vi "CurrentTaskName Request.vi"(8 "error in (no error)":errorcluster, 11 "BuildWorker in":refnum<class "BuildWorker.lvclass">) -> (0 "error out":errorcluster, 3 "BuildWorker out":refnum<class "BuildWorker.lvclass">)   [LabVIEW 2017, in "BuildWorker.lvlib" / "BuildWorker.lvclass"]
uses:
  BuildWorker.lvclass
  BuildWorker.lvclass/BuildWorker.ctl
  WebSocket Server/Actors/WebSocket Client/WebSocket Client Messages/Send Message Msg/Send Message Msg.lvclass/Send Message Msg.ctl
  <vilib>/ActorFramework/Message Enqueuer/Message Enqueuer.lvclass/Message Enqueuer.ctl
  <vilib>/ActorFramework/Message Enqueuer/Enqueue.vi
  WebSocket Server/Actors/WebSocket Client/WebSocket Client Messages/Send Message Msg/Send Message Msg.lvclass
  Applications/National Instruments/LabVIEW 2017 64-bit/vi.lib/ActorFramework/Message/Message.lvclass
  <vilib>/ActorFramework/Message Priority Queue/Priority Enqueue.vi
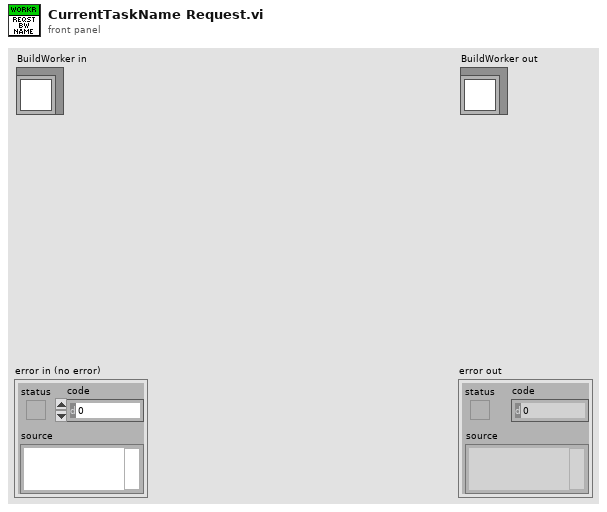
[diagram p1: front panel]
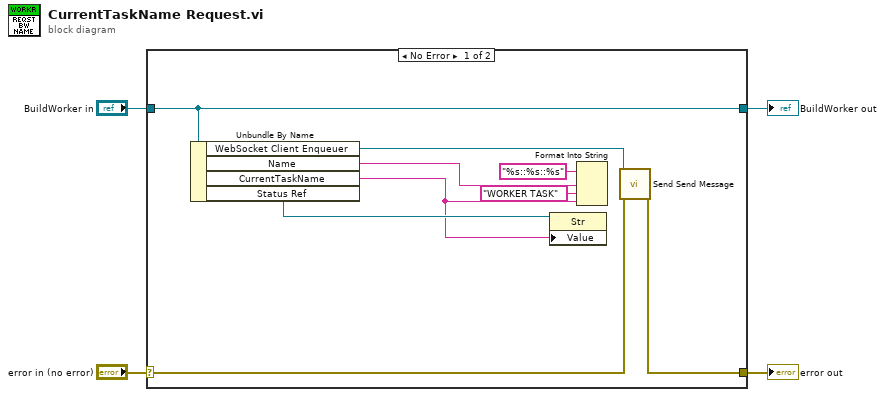
[diagram p0: block diagram]
diagram:
  n1 = case shown="No Error" "error in (no error)" {
    selector: "error in (no error)" -> [w11 w15]
    tunnel: [w10 w15] -> w3
    tunnel: [w13 w14] -> w1
    tunnel: "BuildWorker in" -> [w13 w14]
    frame No Error {
      n2 = Unbundle By Name(w13) -> ("WebSocket Client Enqueuer"=w12:refnum<class "Message Enqueuer.lvclass">, "Name"=w7:string, "CurrentTaskName"=w5:string, "Status Ref"=w9:refnum<vi>)
      n3 = property class="Str"(reference=w9, "Value"=w5) -> ()  [unwired: 1 in, 2 out]
      n4 = Format Into String(format string="%s::%s::%s", w7, "WORKER TASK" ("input 2"), w5) -> ()  [unwired: 2 in, 2 out]
      n5 = call "Send Send Message.vi"("error in (no error)"=w11, "Message Enqueuer in"=w12) -> ("error out"=w10:errorcluster)  [unwired: 8 in, 1 out]
    }
    frame Error {
    }
  }
  "error out" <- w3
  "BuildWorker out" <- w1
